vi "pattern search.vi"() -> ()   [LabVIEW 2013]
uses:
  <vilib>/regexp/Match Regular Expression.xnode
panel:
  in  "Transition of top player - experiment 6":i32[](graph)=[0, 4, 0, 4, 0, 4, 0, 4, 0, 3, 0, -2, 3, 0, 4, 0, 4, -4, 0, -1, 0, 4, 2, -2, 0, 1, -4, 1, 0, 1, 0, -3, 3, 0, -1, 2, 0, 1, 0, -4, 0, 3, 0, 3, 0, 4, 0, -2, 0, -2, 2, 0, 4, -4, 0, 4, 0, 4, 0, -1, 0, 3, 0, -4, 0, 4, 0, 2, 0, 2, 0, 3, 0, 4, 0, -4, 0, 1, 0, 4, 0, 1, -4, 0, 4, 0, 4, -4, 1, 0, -4, 4, 0, 2, -2, 2, -2, 2, -1, 0, 4, 0, 2, 0, 4, 0, 2, 0, -4, 0, 4, 0, 1, 0, -1, 0, 1, 0, 3, -2, 0, 2, 0, 2, -2, 0, -4, 0, 1, -4, 1, 0, 2, 0, 3, -2, 0, -1, 0, -1, 0, 3, 0, 4, 0, 1, 0, -3, 0, -1, 1, -4, 0, 4, 0, -1, 0, 1, 0, 3, 0, -3, 0, 3, 0, 4, 0, -4, 4, 0, -4, 0, -4, 0, 2, 0, 4, -4, 0]
  in  "Transition of bottom player - experiment  6":i32[](graph)=[0, 2, 0, 3, 0, 3, 0, 4, 0, 4, 0, 2, 0, 3, 0, -1, 0, 4, -3, 0, 3, 0, 3, 0, 2, 0, 1, -1, 0, 3, -2, 0, 3, -3, 0, -4, 4, 0, 1, 0, 3, 0, 4, 0, 1, 0, -1, 2, 0, -4, 0, 4, 0, 1, 0, 3, 0, -1, 0, 4, 0, 2, 0, 3, 0, 3, 0, 1, 0, 3, 0, 1, 0, 1, 0, 2, 0, 3, 0, 2, 0, 4, 0, 4, 0, 2, 0, 3, 0, 2, -1, 0, 3, -2, 3, 0, -4, 0, 2, 0, -1, 0, 1, 0, 4, -3, 0, 3, 0, 4, 0, 2, 0, 4, 0, 2, 0, -1, 0, 4, 0, 1, 0, 4, 0, 3, 0, 3, -2, 0, 1, 0, 2, 0, 4, -1, 0, 4, 0, 3, -1, 0, 3, 0, 1, 0, 1, -1, 2, 0, 3, -3, 0, -2, 0, 4, 0, 2, -4, 1, 0, -4, 0, 4, 0, 4, -1, 0, 3, 0, 3, -2, 2, -1, 0, 1, 0]
  in  "FY vs TU trans bottom":i32[](graph)=[1, 0, 2, 0, 2, 0, -3, 0, -3, 0, 1, 0, 4, 0, 1, 0, -4, 0, 2, 0, 2, 0, -4, 0, 1, 0, 3, 0, 3, 0, 3, 0, 4, 0, 4, 0, 4, -4, 4, 0, -4, 0, 2, 0, -2, 0, 3, 0, -4, 1, 0, 4, -4, 1, 0, -2, 3, 0, 2, 0, -1, 0, -2, 0, -2, 0, 3, 0, 3, 0, 1, 0, 3, 0, 3, 0, 3, 0, 4, 0, 3, -2, 2, 0, 1, 0, -2, 0, -3, 4, -4, 0, 1, 0, 1, 0, 4, 0, 2, 0, 3, 0, 4, 0, -1, 0, 1, 0, 3, 0, 2, -2, 0, -2, 3, 0, 2, 0, 2, 0, 1, 0, 4, -4, 4, 0, -1, 0, 4, 0, 4, 0, 2, 0, 2, 0, 4, 0, 4, -3, 0, -3, 4, 0, 3, 0, 4, 0, -3, 0, -3, 0, -1, 0, 1, 0, 3, 0, 3, 0, 2, 0, -4, 0, -1, 0, -4, 4, -4, 4, 0, 1, 0, 1, 0, 3, 0, 4, 0, 2, -1, 0, -3, 0, 3, 0, -4, 0, -4, 0, 3, 0, 2, 0, 3, 0, -2, 2, 0, -1, 0, -2, 0, 2, 0, 4, 0, 3, -2, 2, 0, -2, 2, 0, -4, 0, 2, 0, -3, 0, 4, 0, -4, 0, -3, 3, -3, 0, 1, 0, 3, 0, 3, 0, 4, 0, 1, 0, 2, -2, 0, 1, 0, -3, 4, 0, 4, -4, 4, -4, 0]
  in  "FY vs TU trans top":i32[](graph)=[3, 2, 0, 1, 0, 1, -4, 4, -4, 1, 0, 2, 0, 3, 0, 3, 0, -1, 1, 0, 4, 0, 1, -1, 0, 3, -2, 2, 0, 2, 0, -4, 1, 0, 2, 0, 1, 0, -2, 0, 3, 0, 3, 0, 1, -1, 0, 3, 0, -1, 0, 4, 0, 1, 0, 4, 0, -2, 0, 1, -1, 1, 0, 1, 0, 4, 0, -4, 1, 0, 4, -4, 1, 0, -1, 2, 0, 1, 0, 4, 0, 1, 2, -1, 0, -1, 0, 1, 0, 4, -4, 1, 0, -1, 0, 3, 0, 4, 0, 2, 0, 1, 0, 2, 0, -1, 0, 4, 0, 2, 0, -1, 0, -4, 1, 0, 4, 0, 1, 0, 1, -4, 1, 0, 3, 0, 4, 0, 2, 0, 1, 0, 3, 0, 2, 0, 4, 0, 1, 0, -1, 0, -3, 0, 1, 0, 1, 0, 4, 0, -4, 0, -4, 0, -1, 0, 1, 0, 1, -1, 2, 0, 1, 0, -4, 0, 2, -1, 0, 3, 0, 2, 0, -1, 1, 0, 2, 0, 3, 0, 1, -1, 0, 3, 0, 1, 0, 1, -4, 0, 4, -4, 1, 0, 1, 0, 3, 0, 2, 0, 1, 0, -4, 4, -4, 1, 0, 1, 0, -1, 0, -4, 4, -4, 1, 0, -3, 0, 4, -4, 1, 0, 1, 0, 4, 0, 2, 0, -2, 0, 1, 0, 3, 0, 3, -2, 2, 0, 2, -1, 1, 0, -1, 0, 1, 0, 2, 0, -2, 0, -1, 1, 0, 4, 0, -1, 0, -1, -2, 2, 0, 4, 0, 1, 0, 4, 0, 4, 0, 2, 0]
  out "Array 3":string[][](array[string])
  in  "ChongWei vs LinDan (all england  trans top":i32[](graph)=[3, 1, 0, -4, 4, 0, 1, 0, 2, 0, -2, 2, 0, 2, 0, -2, 3, 0, 1, 0, 4, 0, 2, -1, 0, 1, 0, 1, -1, 0, 4, 0, 4, -4, 0, -1, 0, -4, 4, 0, 2, 0, 1, 0, 4, 0, -2, 3, -2, 2, 0, 2, 0, 1, 0, 2, 0, 3, -2, 0, 2, 0, -1, 0, -2, 3, -2, 0, 1, 0, 4, 0, -2, 2, 0, 3, 0, -3, 0, 1, 0, -2, 3, 0, 3, 0, 3, 0, 3, 0, 3, 0, 3, -2, 2, -2, 3, -2, 3, 0, 3, 0, 4, 0, 2, -1, 0, 2, 1, 0, 4, 0, 2, -1, 0, -4, 4, 0, 1, 0, 2, 0, -1, 2, 0, 2, 0, 1, 0, 1, 0, 3, 0, -2, 3, 0, 1, 0, 1, 0, 4, -4, 1, 0, 3, 0, 2, 0, 1, 0, 3, 0, -2, 2, 0, -1, 1, -1, 0, 2, 0, -4, 0, 2, 0, 2, 0, 2, 0, 2, 0, 4, 0, 1, -1, 2, 1, 0, -1, 0, -2, 3, 0, 2, 0, -4, 0, 1, 0, 1, 0, 1, 0, 2, -1, 0, 2, 0, 4, 0, 1, -1, 0, 1, 0, 2, 0, 4, 0, 2, 0, 3, -2, 2, 0, 3, 0, 3, 0, 4, 0, 2, 0, -2, 0, 4, -4, 0, -1, 2, 0, -4, 4, 0, 3, 0, -4, 1, 0, 1, 0, -1, 1, 0, 2, -2, 3, 0, -2, 0, -1, 0, -2, 1, 0, 4, 0, 1, 0, 2, 0, -2, 0, -2, 3, -2, 2, 0, 2, 0, 2, 0, 1, 0, -3, 0, 2, 0, -2, 3, 0, 1, 0, 1, 0, 4, 0, 1, 0, 3, 0, -2, 0, -2, 3, 0, 1, -4, 0, -1, 2, 0, -1, 0, 1, 0, -4, 0, -2, 2, -2, 2, 0, 2, 0, -4, 0, 1, 0, 2, 0, 3, 0, -1, 0, -2, 0, 4, 0, 4, 0, 2, -2, 0, -4, 0, -4]
  in  "ChongWei vs LinDan (all england  trans bottom":i32[](graph)=[1, 0, 3, 0, 3, 0, -1, 0, 4, 0, 4, 0, 4, -3, 0, 2, 0, 1, 0, -3, 0, 2, 0, 2, 0, -2, 0, 3, 0, -4, 0, -3, 3, 0, 4, 0, 2, 0, 4, 0, -4, 4, 0, 1, 0, 1, -1, 0, -4, 0, 4, 0, -2, 0, -2, 0, 1, 0, 4, -3, 0, 4, -4, 0, 4, 0, 4, 0, 4, 0, 4, 0, 4, -3, 0, 1, 0, 4, 0, 4, 0, 3, 0, 1, 0, 4, 0, -3, 0, -4, 0, -3, 3, 0, -2, 0, 2, 0, 3, 0, 1, 0, 4, 0, 2, 0, 4, 0, 2, 0, 4, 0, 4, 0, 2, 0, 3, 0, 3, 0, 3, 0, -4, 0, -1, 0, 3, 0, 4, 0, -4, 0, -2, 2, 0, 4, 0, 4, 0, 1, 0, -2, 0, -2, 0, -1, 1, 0, -3, 0, 4, 0, 4, 0, 3, 0, 3, 0, -2, 0, 3, 0, 1, 0, -3, 0, 2, 0, 4, 0, 4, 0, 4, 0, 3, 0, 4, 0, 1, 0, 4, 0, -2, 3, 0, 1, 0, 4, -4, 0, 3, 0, -4, 4, 0, 4, -3, 0, 3, 0, 1, 0, 3, 0, 2, 0, 3, 0, 3, 0, 3, -2, 3, -3, 0, 1, 0, 4, 0, 4, 0, 1, 0, -2, 0, 4, 0, 1, 0, 4, 0, 3, 0, 4, 0, -4, 0, 3, -1, 0, -4, 0, 2, 0, -4, 0, 2, 0, 2, 0, 3, 0, 3, 0, 3, 0, 3, 0, 3, 0, 2, 0, -4, 4, 0, 4, 0, 2, -1, 0, -3, 0, -3, 0, 2, 0, 3, 0, -2, 0, 3, 0, -3, 3, -3, 0, -2, 3, 0, 3, 0, 4, -3, 0, 4, -4, 1, 0, 3, 0, 1, 0, 3, 0]
  in  "ChenJin vs DuPengYu ( trans top 2":i32[](graph)=[0, 3, 0, 1, 0, 3, 0, -3, 0, -4, 1, 0, 2, 0, -1, 0, 3, 0, 1, 0, 4, -4, 0, -1, 0, 2, 0, 3, 0, 4, -4, 4, -4, 0, -1, 0, -4, 0, -2, 2, -2, 0, -1, 1, -4, 1, 0, 1, 0, -1, 0, -4, 0, 2, 0, 4, 0, 1, 0, 2, 0, 3, 0, -1, 0, -4, 1, 0, -4, 0, 2, 0, -4, 1, 0, 1, 0, 2, 0, 2, 0, 3, 0, 2, 0, 4, 0, 2, 0, 1, 0, 1, 0, 4, -4, 0, 3, -2, 0, 2, 0, 3, 0, 3, 0, -4, 1, 0, -2, 3, -2, -1, 0, 3, 0, 4, 0, -4, 4, 0, 4, 0, -4, 1, -1, 0, 4, 0, 2, -2, 0, -4, 1, -4, 0, -3, 0, -4, 0, -4, 0, -1, 0, 4, -4, 2, 0, 3, 0, 2, 0, 4, -4, 4, 0, 1, 0, 1, 0, 4, 0, 1, 0, 3, -2, 0, 4, 0, 4, 0, 2, 0, 4, 0, 1, 0, 4, 0, 2, -2, 0, 3, 0, 3, 0, -4, 1, 0, 4, 0, 3, 0, 1, 0, 4, 0, 2, 0, -4, 4, 0, 3, 0, 2, 0, 3, 0, 1, 0, 4, 0, -3, 3, 0, -2, 0, -3, 0, 3, 0]
  in  "ChenJin vs DuPengYu  trans bottom":i32[](graph)=[2, 0, 3, -3, 4, -4, 0, 3, 0, 3, 0, 3, 0, 4, 0, -4, 0, 4, -3, 0, 3, 0, 1, 0, 3, 0, 4, 0, 2, 0, -2, 3, 0, 3, 0, 1, 0, -4, 0, 3, 0, 3, 0, -3, 4, 0, -3, 4, 0, -2, 0, -3, 0, 4, 0, 3, 0, 3, -3, 0, 4, 0, 4, -3, 0, 1, 0, 2, 0, 3, 0, 4, -3, 0, 3, 0, 4, 0, 3, 0, -2, 0, 4, 0, 2, 0, -4, 0, -4, 0, 3, 0, 4, 0, 2, 0, 4, 0, -3, 4, -3, 0, 4, 0, 4, 0, 3, 0, 3, 0, 3, 0, 4, 0, 2, 0, 4, -4, 4, -3, 0, 2, 0, 4, 0, 2, 0, -3, 3, 0, -2, 0, 4, 0, -4, 1, 0, 3, 0, 2, 0, 4, -4, 1, -4, 0, -4, 0, 2, 0, 3, 0, 1, 0, 3, 0, 3, 0, 1, 0, 1, 0, 4, -4, 4, 0, 3, 0, -3, 4, 0, 3, 0, -4, 0, 1, 0, 4, 0, 3, 0, 4, 0, 3, 0]
  in  "Chen jin vs Hu Yun trans bottom 2":i32[](graph)=[0, 2, 0, 3, 0, 3, 0, 4, 0, 4, 0, 2, 0, 3, 0, -1, 0, 4, -3, 0, 3, 0, 3, 0, 2, 0, 1, -1, 0, 3, -2, 0, 3, -3, 0, -4, 4, 0, 1, 0, 3, 0, 4, 0, 1, 0, -1, 2, 0, -4, 0, 4, 0, 1, 0, 3, 0, -1, 0, 4, 0, 2, 0, 3, 0, 3, 0, 1, 0, 3, 0, 1, 0, 1, 0, 2, 0, 3, 0, 2, 0, 4, 0, 4, 0, 2, 0, 3, 0, 2, -1, 0, 3, -2, 3, 0, -4, 0, 2, 0, -1, 0, 1, 0, 4, -3, 0, 3, 0, 4, 0, 2, 0, 4, 0, 2, 0, -1, 0, 4, 0, 1, 0, 4, 0, 3, 0, 3, -2, 0, 1, 0, 2, 0, 4, -1, 0, 4, 0, 3, -1, 0, 3, 0, 1, 0, 1, -1, 2, 0, 3, -3, 0, -2, 0, 4, 0, 2, -4, 1, 0, -4, 0, 4, 0, 4, -1, 0, 3, 0, 3, -2, 2, -1, 0, 1, 0, 4, 0, 2, 0]
  out "Array 2":string[][](array[string])
  in  "ChenJin vs DuPengYu ( trans top":i32[](graph)=[0, 3, 0, 1, 0, 3, 0, -3, 0, -4, 1, 0, 2, 0, -1, 0, 3, 0, 1, 0, 4, -4, 0, -1, 0, 2, 0, 3, 0, 4, -4, 4, -4, 0, -1, 0, -4, 0, -2, 2, -2, 0, -1, 1, -4, 1, 0, 1, 0, -1, 0, -4, 0, 2, 0, 4, 0, 1, 0, 2, 0, 3, 0, -1, 0, -4, 1, 0, -4, 0, 2, 0, -4, 1, 0, 1, 0, 2, 0, 2, 0, 3, 0, 2, 0, 4, 0, 2, 0, 1, 0, 1, 0, 4, -4, 0, 3, -2, 0, 2, 0, 3, 0, 3, 0, -4, 1, 0, -2, 3, -2, -1, 0, 3, 0, 4, 0, -4, 4, 0, 4, 0, -4, 1, -1, 0, 4, 0, 2, -2, 0, -4, 1, -4, 0, -3, 0, -4, 0, -4, 0, -1, 0, 4, -4, 2, 0, 3, 0, 2, 0, 4, -4, 4, 0, 1, 0, 1, 0, 4, 0, 1, 0, 3, -2, 0, 4, 0, 4, 0, 2, 0, 4, 0, 1, 0, 4, 0, 2, -2, 0, 3, 0, 3, 0, -4, 1, 0, 4, 0, 3, 0, 1, 0, 4, 0, 2, 0, -4, 4, 0, 3, 0, 2, 0, 3, 0, 1, 0, 4, 0, -3, 3, 0, -2, 0, -3, 0, 3, 0]
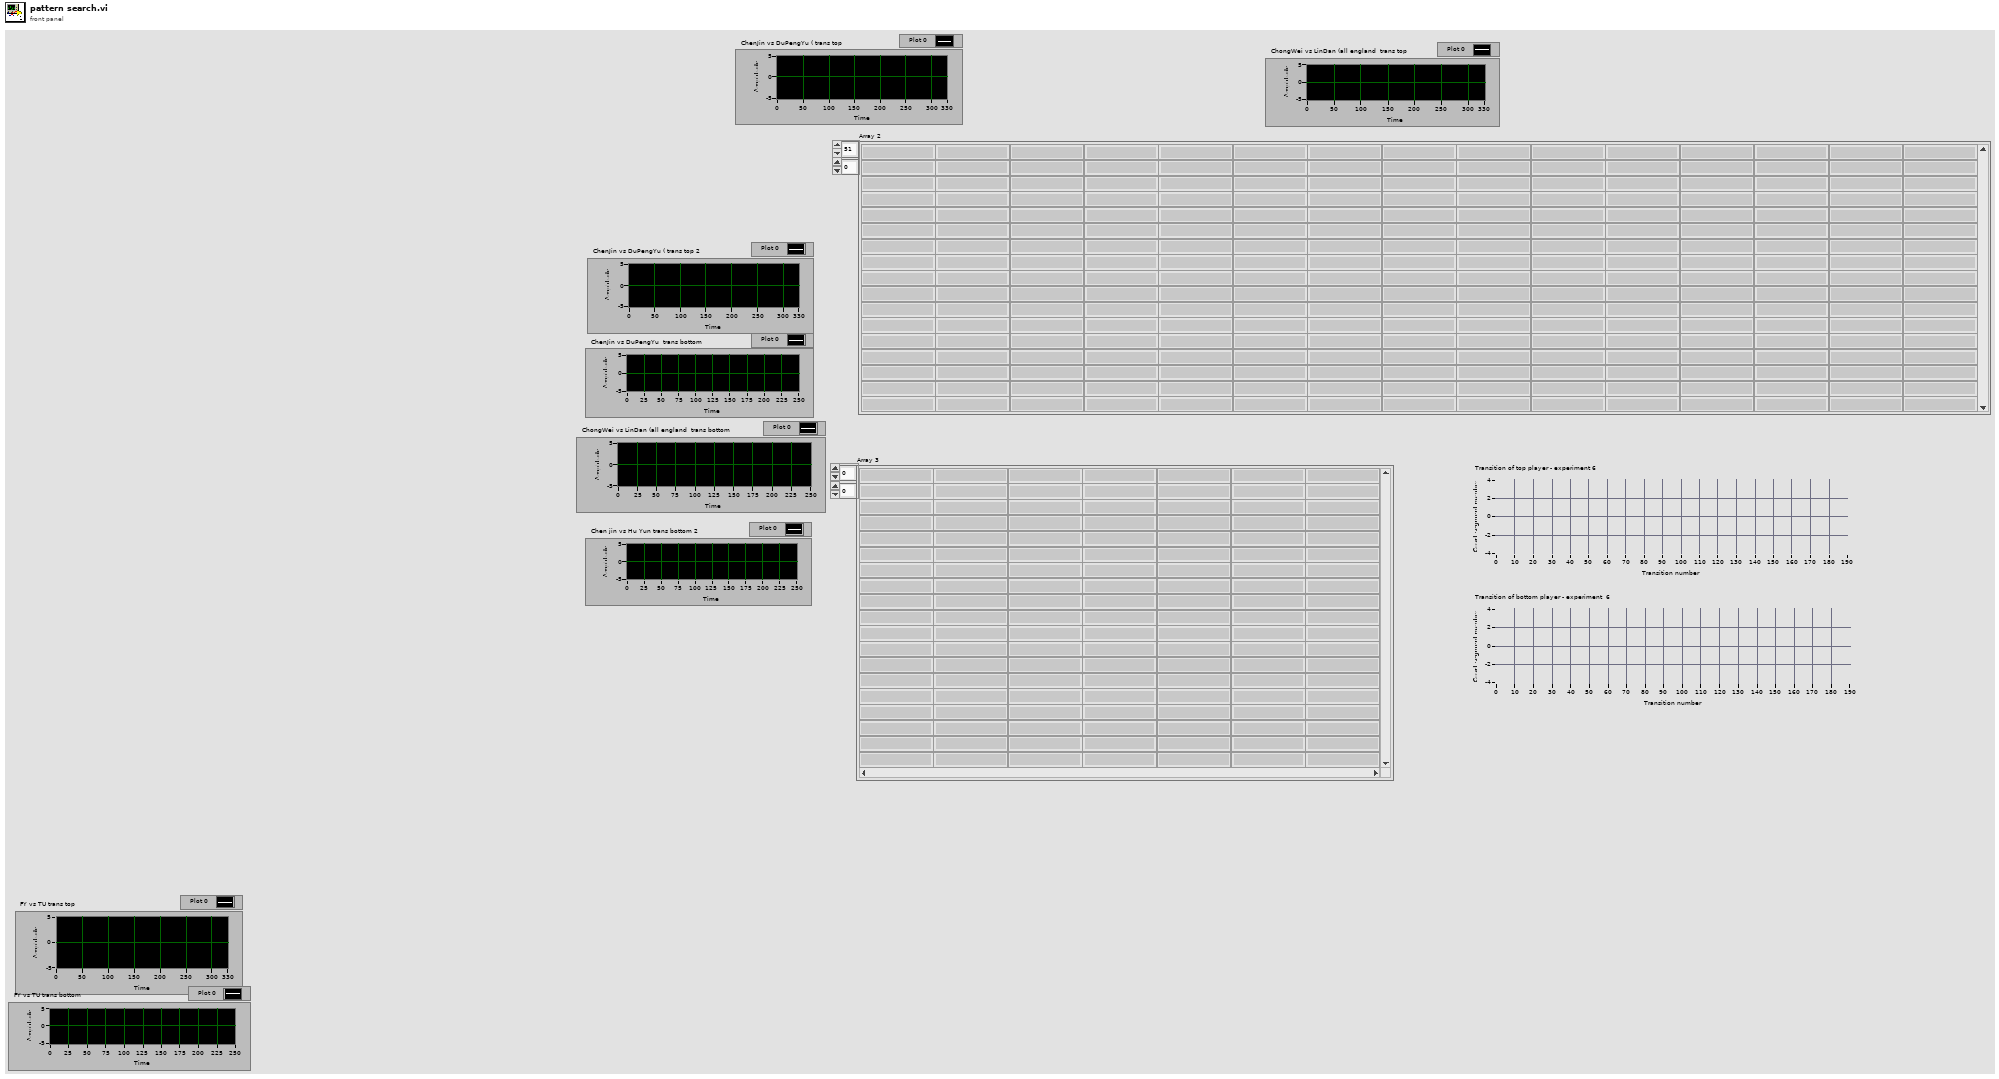
[diagram p1: front panel]
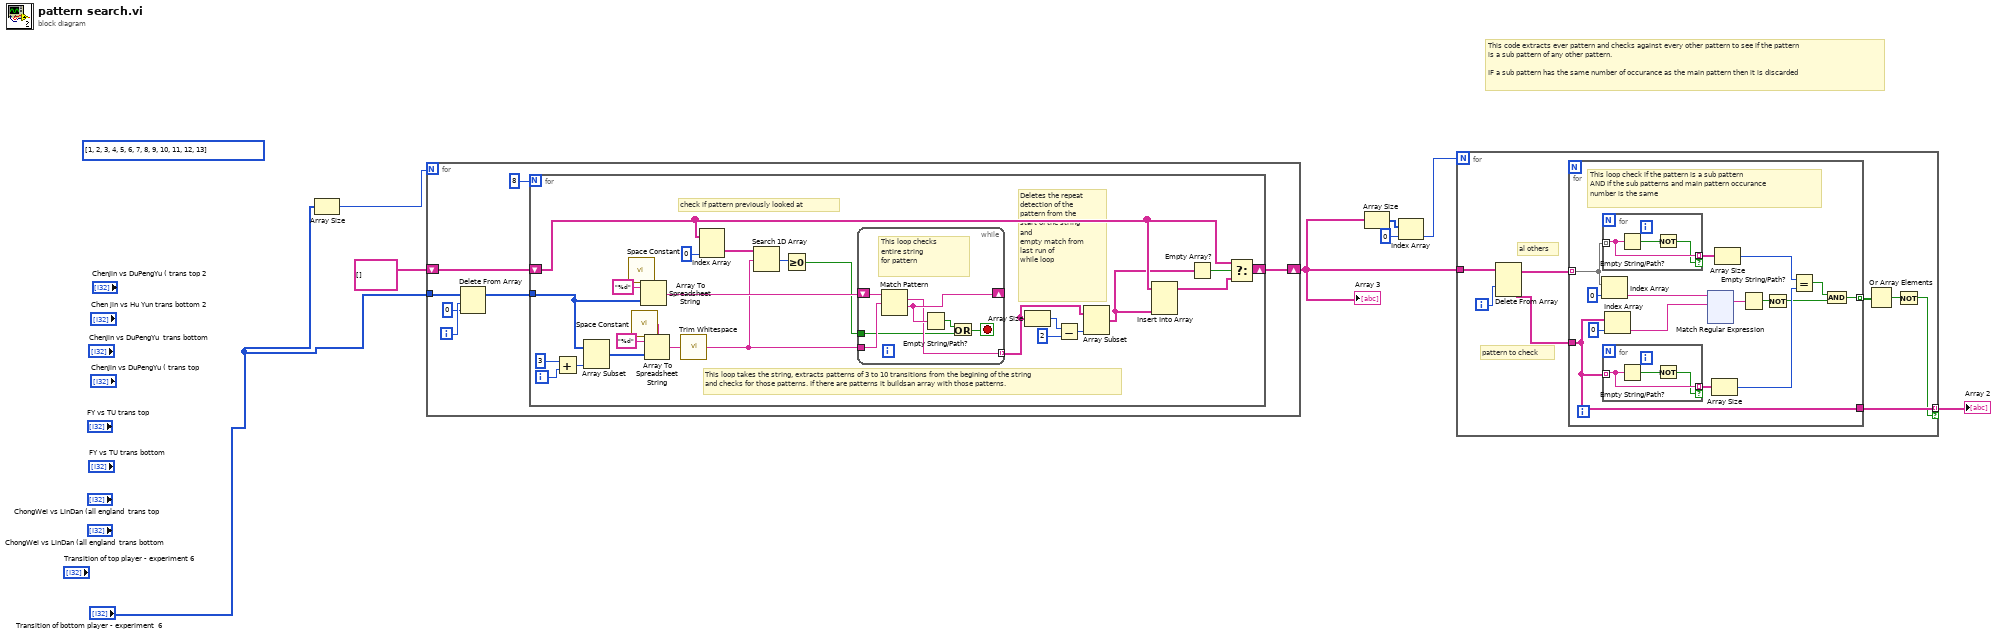
[diagram p0: block diagram]
diagram:
  (unwired) i32[] [1, 2, 3, 4, 5, 6, 7, 8, 9, 10, 11, 12, 13]
  # "This code extracts ever pattern and checks against every other pattern to see if the pattern \nis a sub pattern of any other pattern. \n\nIF a sub pattern has the same number of occurance as the main pattern then it is discarded"
  n1 = Array Size(array="Transition of bottom player - experiment  6") -> (size(s)=w7:i32)
  n2 = for {
    N: w7 -> [_]
    tunnel: "Transition of bottom player - experiment  6" -> [w11]
    shift-right: [w14] -> w2
    shift-left: string[][] [] -> [w13]
    i -> [w12]
    n3 = Delete From Array(array=w11, length=w12, index=0) -> (array with subset deleted=w10:i32[])  [unwired: 1 out]
    n4 = for {
      N: 8 ("length") -> [_]
      tunnel: w10 -> [w34]
      shift-right: [w25] -> w14
      shift-left: w13 -> [w23]
      i -> [w32]
      # "Deletes the repeat detection of the \npattern from the start of the string and\nempty match from last run of \nwhile loop"
      # "check if pattern previously looked at"
      # "This loop takes the string, extracts patterns of 3 to 10 transitions from the begining of the string\nand checks for those patterns. If there are patterns it buildsan array with those patterns."
      n5 = Add(x=3, y=w32) -> (x+y=w30:i32)
      n6 = Array Subset(array=w34, length=w30) -> (w38:i32[])  [unwired: 1 in]
      n7 = call <vilib>:"Space Constant.vi"() -> ("String"=w36:string)
      n8 = call <vilib>:"Space Constant.vi"() -> ("String"=w40:string)
      n9 = Array To Spreadsheet String(delimiter (Tab)=w36, array=w34, 3:"%d" ("format string")) -> (spreadsheet string=w35:string)
      n10 = Array To Spreadsheet String(delimiter (Tab)=w40, array=w38, 3:"%d" ("format string")) -> (spreadsheet string=w33:string)
      n11 = call <vilib>:"Trim Whitespace.vi"("string"=w33) -> ("trimmed string"=w20:string)  [unwired: 1 in]
      n12 = Index Array(array=w23, index (col)=0 ("disabled index (col)")) -> (element=w21:string[])  [unwired: 1 in]
      n13 = Search 1D Array(1D array=w21, element=w20) -> (index of element=w19:i32)  [unwired: 1 in]
      n14 = Greater Or Equal To 0?(x=w19) -> (x >= 0?=w18:bool)
      n15 = while {
        tunnel: w20 -> [w46]
        shift-right: [w45] -> _
        shift-left: w35 -> [w47]
        tunnel: [w44] -> w17 mode=indexing
        tunnel: w18 -> [w41]
        stop <- w43 stop-if-true
        # "This loop checks\nentire string\nfor pattern"
        n16 = Match Pattern(string=w47, regular expression=w46) -> (match substring=w44:string, after substring=w45:string)  [unwired: 1 in, 2 out]
        n17 = Empty String/Path?(string/path=w45) -> (empty?=w42:bool)
        n18 = Or(x=w42, y=w41) -> (x .or. y?=w43:bool)
      }
      n19 = Array Size(array=w17) -> (size(s)=w29:i32)
      n20 = Subtract(x=w29, y=2) -> (x-y=w27:i32)
      n21 = Array Subset(array=w17, length=w27) -> (w16:string[])  [unwired: 1 in]
      n22 = Insert Into Array(array=w23, new element=w16) -> (w24:string[][])  [unwired: 2 in]
      n23 = Empty Array?(array=w16) -> (empty?=w26:bool)
      n24 = Select(t=w23, s=w26, f=w24) -> (s? t:f=w25:string[][])
    }
  }
  "Array 3" <- w2
  n25 = Array Size(array=w2) -> (size(s)=w6:i32[])
  n26 = Index Array(array=w6, index=0) -> (element=w4:i32)
  n27 = for {
    N: w4 -> [_]
    tunnel: w2 -> [w55]
    tunnel: [w51] -> w3 mode=indexing if=w48
    i -> [w54]
    # "al others"
    # "pattern to check"
    n28 = Delete From Array(array=w55, index (row)=w54) -> (deleted portion=w52:string[], array with subset deleted=w53:string[][])  [unwired: 2 in]
    n29 = for {
      tunnel: w53 -> [w61] mode=indexing
      tunnel: w52 -> [w57]
      tunnel: [w62] -> w50 mode=indexing
      tunnel: [w57] -> w51
      # "This loop check if the pattern is a sub pattern \nAND if the sub patterns and main pattern occurance \nnumber is the same"
      n30 = Index Array(array=w61, index=0) -> (element=w69:string)
      n31 = for {
        tunnel: w61 -> [w76] mode=indexing
        tunnel: [w76] -> w60 mode=indexing if=w74
        n32 = Empty String/Path?(string/path=w76) -> (empty?=w75:bool)
        n33 = Not(x=w75) -> (.not. x?=w74:bool)
      }
      n34 = for {
        tunnel: w57 -> [w73] mode=indexing
        tunnel: [w73] -> w59 mode=indexing if=w71
        n35 = Empty String/Path?(string/path=w73) -> (empty?=w72:bool)
        n36 = Not(x=w72) -> (.not. x?=w71:bool)
      }
      n37 = Index Array(array=w57, index=0) -> (element=w56:string)
      n38 = xnode "Match Regular Expression"("input string"=w69, "regular expression"=w56) -> ("whole match"=w66:string)  [unwired: 4 in, 4 out]
      n39 = Array Size(array=w59) -> (size(s)=w67:i32)
      n40 = Array Size(array=w60) -> (size(s)=w68:i32)
      n41 = Empty String/Path?(string/path=w66) -> (empty?=w65:bool)
      n42 = Not(x=w65) -> (.not. x?=w63:bool)
      n43 = Equal?(x=w68, y=w67) -> (x = y?=w64:bool)
      n44 = And(x=w64, y=w63) -> (x .and. y?=w62:bool)
    }
    n45 = Or Array Elements(Boolean array=w50) -> (logical OR=w49:bool)
    n46 = Not(x=w49) -> (.not. x?=w48:bool)
  }
  "Array 2" <- w3
